vi "arrayerrculster.vi"(1 "Array In":errorcluster[](array[cluster])) -> (0 "Array Out":errorcluster[](array[cluster]))   [LabVIEW 2013]
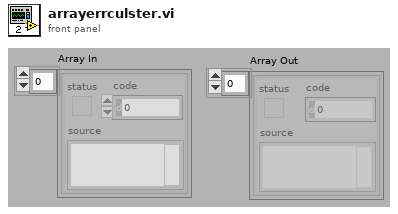
[diagram p1: front panel]
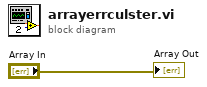
[diagram p0: block diagram]
diagram:
  "Array Out" <- "Array In"
